vi "uTTA_PostProcessing_V2.vi"() -> ()   [LabVIEW 2021]
uses:
  Postprocessing/CTRL_DUT_SETTINGS.ctl
  Postprocessing/uTTA_MetaData.ctl
  <vilib>/Utility/miscctls.llb/LVPointTypeDef.ctl
  7dfeb571-d9df-452e-894a-a3940027d341.vi
  <vilib>/Comparison/Less/Less Functor/Less Functor.lvclass
panel:
  out "RunTime Scale":dbl
  out "Runtime ParseFile":dbl
  out "RunTime ReadFile":dbl
  in  "File Path":path
  out "Updated":bool
  in  "Tab Control":T1(tab)
  in  "CAL_File":path=path "C:/temp/Eigenentwicklungen/Octave_Thermal_Modelling/Measurement_Data/20221220_uTTA_HW200_CALIBRATION.tdms"
  out "uTTA_MetaData":T2 {"Interpolation Factor m" format="%.2g"; "Interpolation Offset" format="%.2g"; "Chip Size" format="%.2gmm²"; "Heating Power" format="%.3pW"; "Cool Volt Deviation" format="%.3pV"; "Cool Voltage" format="%.3pV"; "Tsamp,fast" format="%#_3gus"; "Tsamp,slow" format="%dus"; "T_Preheat" format="%ds"; "T_Heat" format="%ds"; "T_Cool" format="%ds"}
  in  "First Samples":i32=2000
  in  "Off-Voltage":dbl=0.3 caption="Treshhold" min=-10.0 max=10.0 step=0.01
  out "Off-Voltage Index":i32 caption="Index"
  in  "Cut at Off-Voltage":bool=TRUE caption="Enable"
  out "Heating Power":dbl format="%#_3pW"
  out "Cool Volt Deviation":dbl format="%.1pV"
  out "Cool Voltage":dbl format="%.2pV"
  in  "DUT Settings":T3={"Test Comment"="", "Channel No."="", "Sample No."="", "TSP Offset"=0.0, "TSP Cubic Gain"=0.0, "TSP Linear Gain"=-0.0026} {"TSP Linear Gain" format="%.3pV/K"}
  in  "Filter Signals":bool=TRUE
  out "MeasDataLng":cluster{dbl[], "Diode_Temperature":dbl[]}[](graph)
  out "Meas_scaled":cluster{dbl[], "Diode_Temperature":dbl[]}[](graph)
  in  "PlotScale":bool
  out "Interpolation":cluster{dbl[], dbl[]}[](graph)
  out "Factor m":dbl format="%#_6p"
  out "Chip Size":dbl format="%#_6f mm²"
  out "Offset":dbl
  in  "Export":bool
  out "CoolingCurve":cluster{"Time":dbl[], "delta_T":dbl[]}[](graph)
  out "RunTime":dbl format="%#_3gs"
  in  "Exit":bool
  in  "Update":bool
  # "Filtering"
  # "Pre-Heating Cold Voltage"
  # "Off-Voltage curve cutting"
  # "Cooling curve extrapolation"
  # "Heating Power"
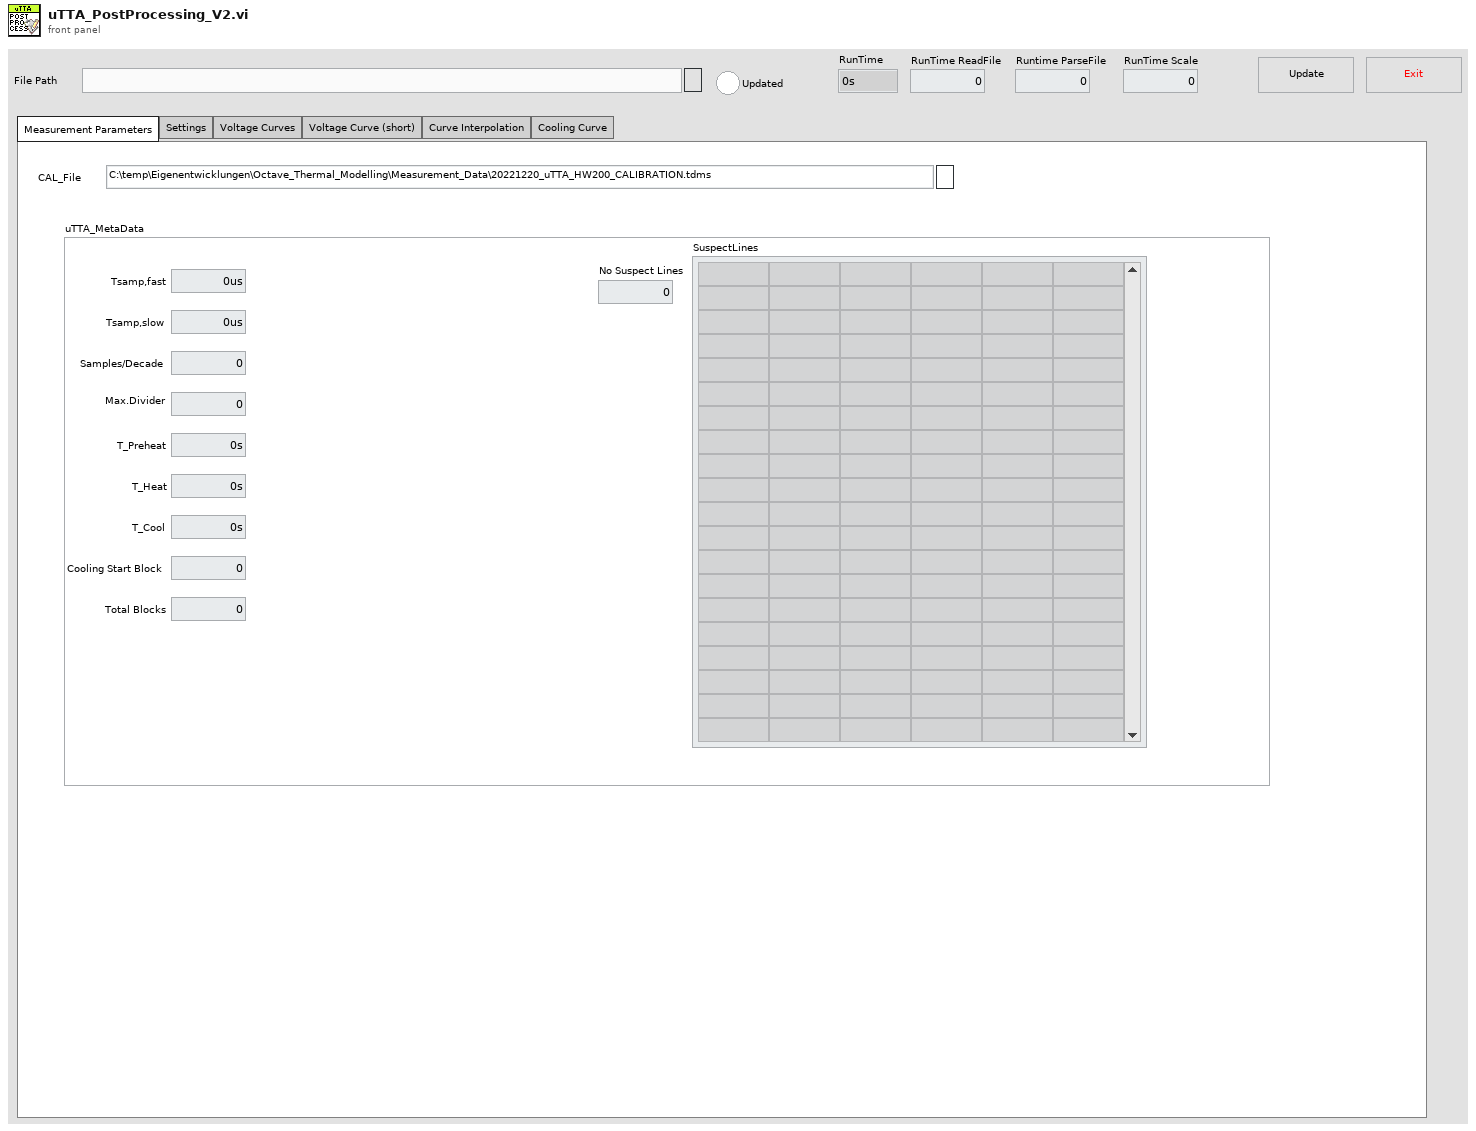
[diagram p1: front panel]
types:
  T1 = enum32{"Measurement Parameters", "Settings", "Voltage Curves", "Voltage Curve (short)", "Curve Interpolation", "Cooling Curve"}
  T2 = typedef "uTTA_MetaData.ctl" = cluster{"Tsamp,fast":dbl, "Tsamp,slow":dbl, "Samples/Decade":u32, "Max.Divider":u32, "T_Preheat":dbl, "T_Heat":dbl, "T_Cool":dbl, "Cooling Start Block":u32, " Total Blocks":u32, "SuspectLines":string[][], "Cool Voltage":dbl, "Cool Volt Deviation":dbl, "Heating Power":dbl, "Chip Size":dbl, "Interpolation Offset":dbl, "Interpolation Factor m":dbl, "No Suspect Lines":u32}
  T3 = typedef "CTRL_DUT_SETTINGS.ctl" = cluster{"Test Comment":string, "Channel No.":string, "Sample No.":string, "TSP Offset":dbl, "TSP Cubic Gain":dbl, "TSP Linear Gain":dbl}
  T4 = typedef "LVPointTypeDef.ctl" = cluster{"Horizontal":i16, "Vertical":i16}
  T5 = enum16{"open", "replace", "create", "open or create", "replace or create", "replace or create with confirmation"}
  T6 = typedef "LVCursorListTypeDef.ctl" = cluster{"Name":string, "Color":u32, "Style":u8, "Point Style":u8, "Name Visible":bool, "Allow Drag":bool, "Cursor Mode":u32, "Plot":i32, "Index":i32, "Position":cluster{"X":dbl, "Y":dbl}, "X Scale":u32, "Y Scale":u32, "Watch Plots":i32[], "Watch All Plots":bool, "Plot Area":i32, "Label Offset":cluster{"X":dbl, "Y":dbl}}[]
  T7 = cluster{"Name":string, "Color":u32, "Style":u8, "Point Style":u8, "Name Visible":bool, "Allow Drag":bool, "Cursor Mode":u32, "Plot":i32, "Index":i32, "Position":cluster{"X":dbl, "Y":dbl}, "X Scale":u32, "Y Scale":u32, "Watch Plots":i32[], "Watch All Plots":bool, "Plot Area":i32, "Label Offset":cluster{"X":dbl, "Y":dbl}}
  T8 = typedef "CTL_uTTA_MeasurementDataValues.ctl" = cluster{"BlockNo":i32[], "ADC":i32[][], "PGA":i32[], "Thermocouple":dbl[][]}
  T9 = typedef "CTL_uTTA_MeasurementData.ctl" = cluster{"Time":dbl[], "Voltage":dbl[], "Current":dbl[], "delta_T":dbl[], "T_ext":dbl[][]}
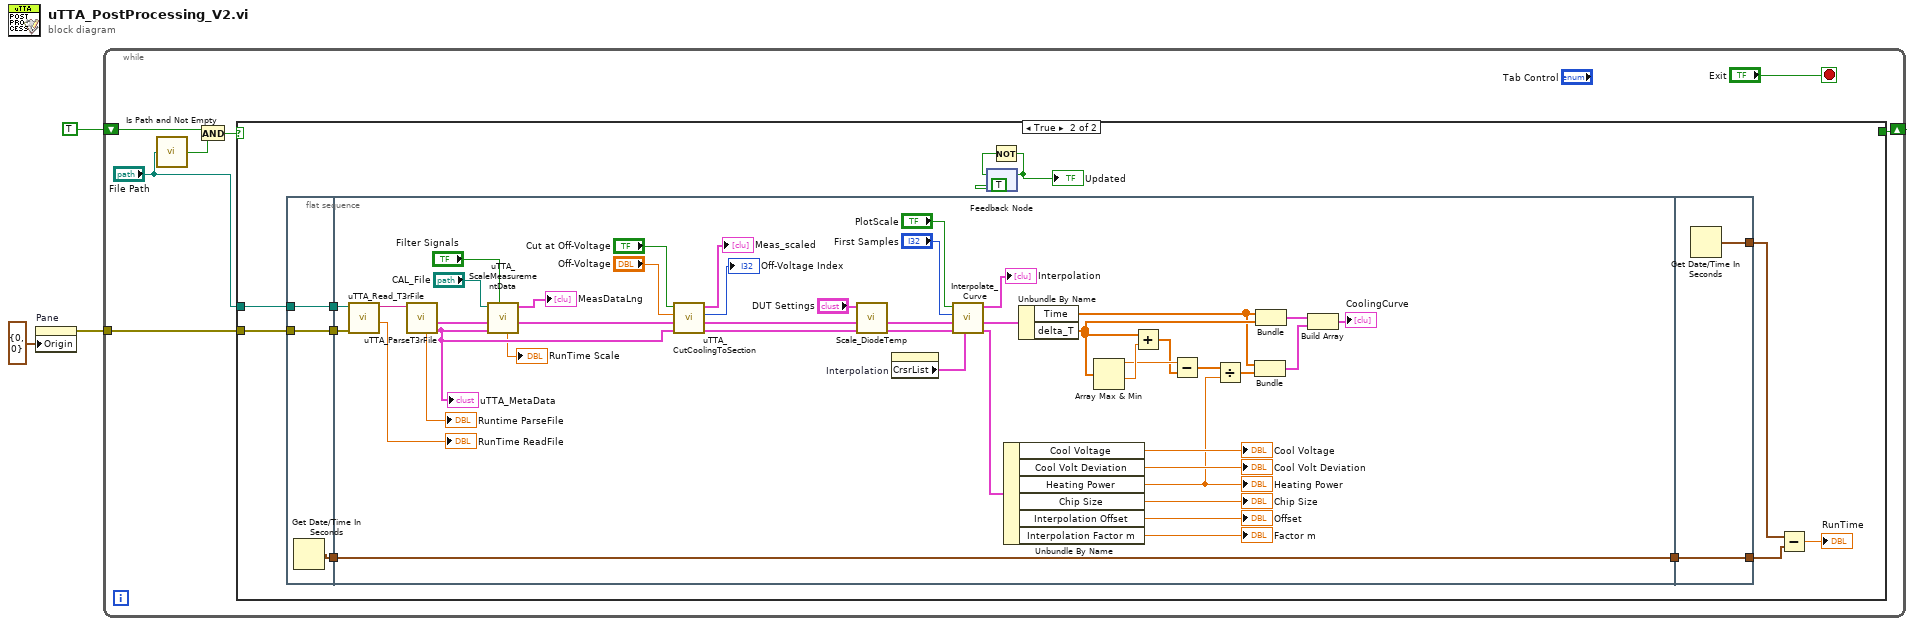
[diagram p0: block diagram]
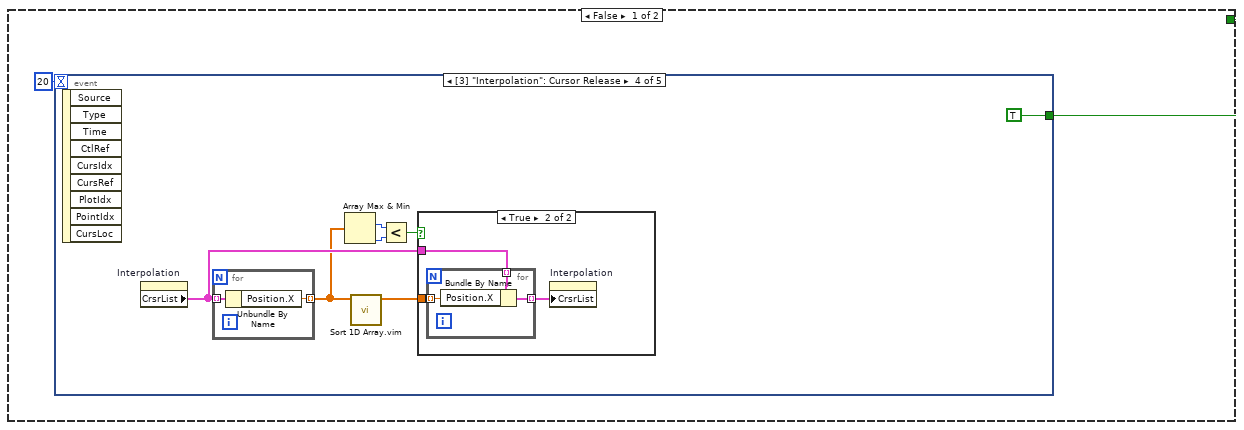
[diagram p2: hidden frame]
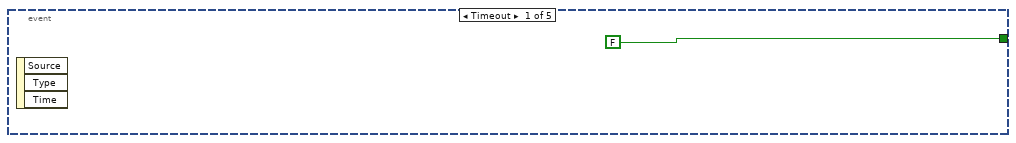
[diagram p3: hidden frame]
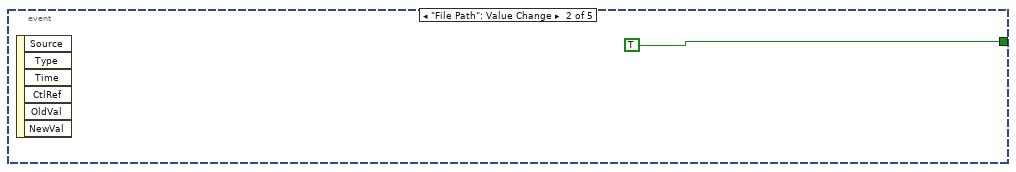
[diagram p4: hidden frame]
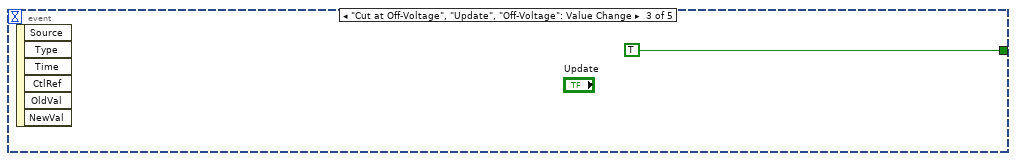
[diagram p5: hidden frame]
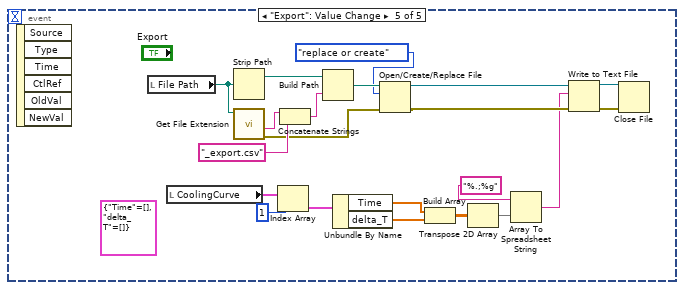
[diagram p7: hidden frame]
diagram:
  n1 = property on="Pane" class="Pane"("Origin"=T4 {"Horizontal"=0, "Vertical"=0}) -> (error out=w2:errorcluster)  [unwired: 2 in, 1 out]
  n2 = while {
    tunnel: w2 -> [w9]
    shift-right: [w5] -> _
    shift-left: TRUE ("Update") -> [w6]
    stop <- "Exit" stop-if-true
    n3 = call <vilib>:"Is Path and Not Empty.vi"("path"="File Path") -> ("Is Path and Not Empty?"=w7:bool)  [unwired: 4 in]
    n4 = And(x=w6, y=w7) -> (x .and. y?=w4:bool)
    n5 = case shown="True" w4 {
      tunnel: w9 -> [_ w56]
      tunnel: "File Path" -> [_ w53]
      tunnel: [w11 _] -> w5
      frame False {
        n6 = event shown="[3] \"Interpolation\": Cursor Release" {
          selector: _ -> [_ _ _ _ _]
          dyn-events: _ -> [_ _ _ _ _]
          timeout: 20 -> [_ _ _ _ _]
          tunnel: [FALSE ("Update") TRUE ("Update") TRUE ("Update") TRUE ("Update") _] -> w11
          event Timeout {
            n7 = event-data() -> ()  [unwired: 1 in, 3 out]
          }
          event "File Path": Value Change {
            n8 = event-data() -> ()  [unwired: 1 in, 6 out]
          }
          event "Cut at Off-Voltage", "Update", "Off-Voltage": Value Change {
            n9 = event-data() -> ()  [unwired: 1 in, 6 out]
          }
          event "Interpolation": Cursor Release {
            n10 = event-data() -> ()  [unwired: 1 in, 9 out]
            n11 = property on="Interpolation" class="XYGraph (strict)"() -> ("CrsrList"=w22:T6)  [unwired: 2 in, 2 out]
            n12 = for {
              tunnel: w22 -> [w30] mode=indexing
              tunnel: [w29] -> w20 mode=indexing
              n13 = Unbundle By Name(w30) -> ("Position.X"=w29:dbl)
            }
            n14 = Array Max & Min(array=w20) -> (max index (indices)=w19:i32, min index (indices)=w18:i32)  [unwired: 2 out]
            n15 = call "Sort 1D Array.vim"("unsorted array"=w20) -> ("sorted array"=w21:dbl[])  [unwired: 10 in]
            n16 = Less?(x=w19, y=w18) -> (x < y?=w17:bool)
            n17 = case shown="True" w17 {
              tunnel: w22 -> [_ w25]
              tunnel: w21 -> [_ w24]
              frame False {
              }
              frame True {
                n18 = for {
                  tunnel: w25 -> [w28] mode=indexing
                  tunnel: w24 -> [w27] mode=indexing
                  tunnel: [w26] -> w23 mode=indexing
                  n19 = Bundle By Name(cluster=w28, "Position.X"=w27) -> (w26:T7)
                }
                n20 = property on="Interpolation" class="XYGraph (strict)"("CrsrList"=w23) -> ()  [unwired: 2 in, 2 out]
              }
            }
          }
          event "Export": Value Change {
            (unwired) cluster{"Time":dbl[], "delta_T":dbl[]} {"Time"=[], "delta_T"=[]} ("element")
            n21 = event-data() -> ()  [unwired: 1 in, 6 out]
            n22 = local read "File Path"() -> (w51:path)
            n23 = local read "CoolingCurve"() -> (w43:cluster{"Time":dbl[], "delta_T":dbl[]}[])
            n24 = Strip Path(path=w51) -> (stripped path=w48:path)  [unwired: 1 out]
            n25 = call <vilib>:"Get File Extension.vi"("file"=w51) -> ("error out"=w44:errorcluster, "filename without extension"=w50:string)  [unwired: 6 in, 3 out]
            n26 = Index Array(array=w43, index=1) -> (element=w41:cluster{"Time":dbl[], "delta_T":dbl[]})
            n27 = Concatenate Strings(w50, "_export.csv" ("string")) -> (w47:string)
            n28 = Build Path(base path=w48, name or relative path=w47) -> (appended path=w46:path)
            n29 = Unbundle By Name(w41) -> ("Time"=w40:dbl[], "delta_T"=w39:dbl[])
            n30 = Open/Create/Replace File(file path (use dialog)=w46, error in=w44, operation (0:open)=T5."replace or create") -> (refnum out=w38:refnum<file>, error out=w37:errorcluster)  [unwired: 3 in, 1 out]
            n31 = Build Array(w40, w39) -> (w32:dbl[][])
            n32 = Transpose 2D Array(2D array=w32) -> (transposed array=w31:dbl[][])
            n33 = Array To Spreadsheet String(array=w31, 3:"%.;%g" ("format string")) -> (spreadsheet string=w35:string)  [unwired: 1 in]
            n34 = Write to Text File(file (use dialog)=w38, text=w35, error in=w37) -> (refnum out=w33:refnum<file>, error out=w34:errorcluster)  [unwired: 1 in, 1 out]
            n35 = Close File(refnum=w33, error in=w34) -> ()  [unwired: 2 out]
          }
        }
      }
      frame True {
        n36 = flat-sequence {
          tunnel: [w66] -> w57
          tunnel: w56 -> [w65]
          tunnel: [w65] -> w55
          tunnel: w53 -> [w64]
          tunnel: [w64] -> w54
          tunnel: [w80] -> w58
          tunnel: w57 -> [w80]
          tunnel: w55 -> [w79]
          tunnel: w54 -> [w78]
          tunnel: [w111] -> w63
          tunnel: w58 -> [w110]
          tunnel: [w110] -> w52
          frame #0 {
            n37 = Get Date/Time In Seconds() -> (seconds since 1Jan1904=w66:timestamp)
          }
          frame #1 {
            n38 = call "uTTA_Read_T3rFile.vi"("error in"=w79, "File Path"=w78) -> ("RunTime"=→"RunTime ReadFile":dbl, "T3R-File"=w81:string)  [unwired: 7 in, 1 out]
            n39 = call "uTTA_ParseT3rFile.vi"("uTTA_MeasureFile"=w81) -> ("Runtime ParseFile"=→"Runtime ParseFile":dbl, "uTTA_MeasureData"=w98:T8, "uTTA_MetaData"=w107:T2)  [unwired: 6 in]
            "uTTA_MetaData" <- w107
            n40 = call "uTTA_ScaleMeasurementData.vi"("Filter Signals"="Filter Signals", "uTTA_MetaData_in"=w107, "uTTA_MeasureData"=w98, "CAL_File"="CAL_File") -> ("MeasData_out"=w94:T9, "Graph_out"=→"MeasDataLng":cluster{"Array":dbl[], "Array":dbl[]}[], "RunTime Scale"=→"RunTime Scale":dbl)  [unwired: 5 in]
            n41 = call "uTTA_CutCoolingToSection.vi"("uTTA_MetaData"=w107, "MeasData_in"=w94, "Off-Voltage"="Off-Voltage", "Cut at Off-Voltage"="Cut at Off-Voltage") -> ("uTTA_MetaData_out"=w87:T2, "MeasData_out"=w90:T9, "Index"=→"Off-Voltage Index":i32, "Graph_out"=→"Meas_scaled":cluster{"Array":dbl[], "Array":dbl[]}[])
            n42 = call "Scale_DiodeTemp.vi"("uTTA_MetaData_in"=w87, "uTTA_MeasData_in"=w90, "DUT Settings"="DUT Settings") -> ("uTTA_MeasData_out"=w89:T9)  [unwired: 3 in, 1 out]
            n43 = property on="Interpolation" class="XYGraph (strict)"() -> ("CrsrList"=w91:T6)  [unwired: 2 in, 2 out]
            n44 = call "Interpolate_Curve.vi"("Cursor List"=w91, "uTTA_MetaData_in"=w87, "uTTA_MeasData_in"=w89, "First Samples"="First Samples", "PlotScale [SQRT-Sclale]"="PlotScale") -> ("uTTA_MetaData_out"=w88:T2, "uTTA_MeasData_out"=w83:T9, "Plot"=→"Interpolation":cluster{dbl[], dbl[]}[])  [unwired: 2 in]
            n45 = Unbundle By Name(w88) -> ("Cool Voltage"=→"Cool Voltage":dbl, "Cool Volt Deviation"=→"Cool Volt Deviation":dbl, "Heating Power"=w67:dbl, "Chip Size"=→"Chip Size":dbl, "Interpolation Offset"=→"Offset":dbl, "Interpolation Factor m"=→"Factor m":dbl)
            "Heating Power" <- w67
            n46 = Unbundle By Name(w83) -> ("Time"=w76:dbl[], "delta_T"=w77:dbl[])
            n47 = Array Max & Min(array=w77) -> (max value=w71:dbl, min value=w72:dbl)  [unwired: 2 out]
            n48 = Add(x=w77, y=w72) -> (x+y=w70:dbl[])
            n49 = Subtract(x=w71, y=w70) -> (x-y=w69:dbl[])
            n50 = Divide(x=w69, y=w67) -> (x/y=w68:dbl[])
            n51 = Bundle("Time"=w76, w68) -> (w74:cluster{"Time":dbl[], dbl[]})  [unwired: 1 in]
            n52 = Bundle("Time"=w76, "delta_T"=w77) -> (w75:cluster{"Time":dbl[], "delta_T":dbl[]})  [unwired: 1 in]
            n53 = Build Array(w75, w74) -> (→"CoolingCurve":cluster{"Time":dbl[], "delta_T":dbl[]}[])
          }
          frame #2 {
            n54 = Get Date/Time In Seconds() -> (seconds since 1Jan1904=w111:timestamp)
          }
        }
        n55 = feedback #1(TRUE) -> (w61:bool)
        n56 = Not(x=w61) -> (.not. x?=w60:bool)
        "Updated" <- w60
        n57 = feedback-in #1(w60) -> ()
        n58 = Subtract(x=w63, y=w52) -> (x-y=→"RunTime":dbl)
      }
    }
  }
